vi "Try Parse.vi"(0 "SG SC2250 Path in":refnum<class "SG SC2250 Path.lvclass">, 5 "Config Row":string[](array[string]), 11 "error in (no error)":errorcluster) -> (4 "SG SC2250 Path out":refnum<class "SG SC2250 Path.lvclass">, 6 "Is of type?":bool=TRUE, 15 "error out":errorcluster)   [LabVIEW 2023, in "RFFixtureCharact.RFPM.lvlib" / "SG SC2250 Path.lvclass"]
uses:
  SG SC2250 Path.lvclass
  <vilib>/Utility/error.llb/Trim Whitespace One-Sided.vi
  Common/RFCalAndFixtureCharact.Common.lvlib
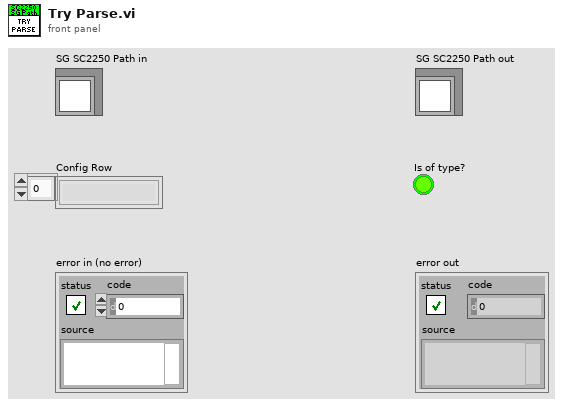
[diagram p1: front panel]
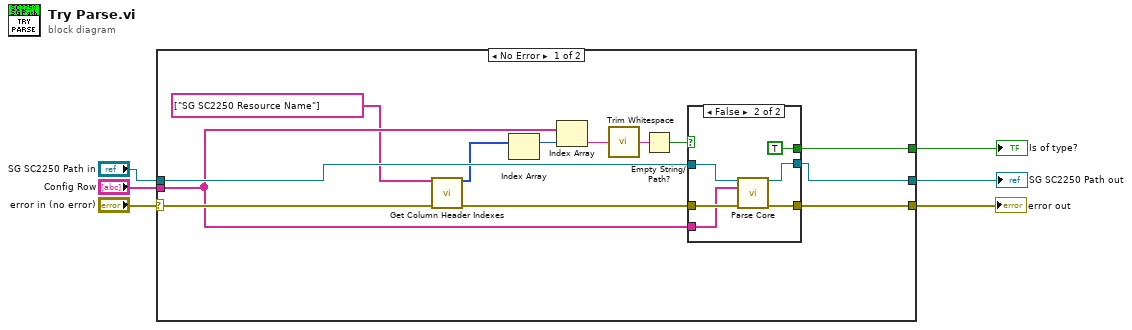
[diagram p0: block diagram]
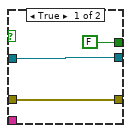
[diagram p2: hidden frame]
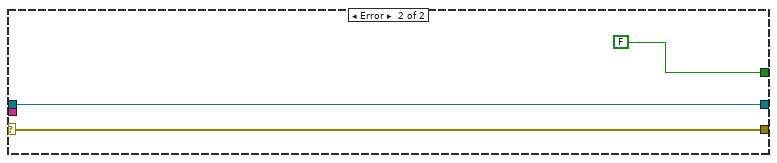
[diagram p3: hidden frame]
diagram:
  n1 = case shown="No Error" "error in (no error)" {
    selector: "error in (no error)" -> [w18 w31]
    tunnel: [w7 w31] -> w4
    tunnel: [w19 FALSE ("Is of type?")] -> w3
    tunnel: [w8 w30] -> w2
    tunnel: "Config Row" -> [w12 _]
    tunnel: "SG SC2250 Path in" -> [w13 w30]
    frame No Error {
      n2 = call "Get Column Header Indexes.vi"("Column Header Names"=string[] ["SG SC2250 Resource Name"], "error in"=w18) -> ("Column Header Indices"=w10:i32[], "error out"=w14:errorcluster)  [unwired: 11 in, 1 out]
      n3 = Index Array(array=w10) -> (element=w9:i32)  [unwired: 1 in]
      n4 = Index Array(array=w12, index=w9) -> (element=w15:string)
      n5 = call <vilib>:"Trim Whitespace.vi"("string"=w15) -> ("trimmed string"=w17:string)  [unwired: 1 in]
      n6 = Empty String/Path?(string/path=w17) -> (empty?=w16:bool)
      n7 = case shown="False" w16 {
        tunnel: [w21 w23] -> w7
        tunnel: w14 -> [w21 w28]
        tunnel: w13 -> [w22 w27]
        tunnel: w12 -> [_ w26]
        tunnel: [FALSE ("Is of type?") TRUE ("Is of type?")] -> w19
        tunnel: [w22 w24] -> w8
        frame True {
        }
        frame False {
          n8 = call-dynamic "Parse Core.vi"("SG SC2250 Path in"=w27, "Config Row"=w26, "error in (no error)"=w28) -> ("SG SC2250 Path out"=w24:refnum<class "SG SC2250 Path.lvclass">, "error out"=w23:errorcluster)  [unwired: 11 in]
        }
      }
    }
    frame Error {
    }
  }
  "error out" <- w4
  "SG SC2250 Path out" <- w2
  "Is of type?" <- w3
